vi "Determine Packet Type.vi"(11 "Packet First Byte":u8 format="%08b") -> (3 "Packet Type":refnum<class "ControlPacket.lvclass">)   [LabVIEW 2013, in "ControlPacket.lvclass"]
uses:
  ControlPacket.lvclass
  CONNECT/CONNECT.lvclass
  CONNACK/CONNACK.lvclass
  PUBLISH/PUBLISH.lvclass
  PUBACK/PUBACK.lvclass
  PUBREC/PUBREC.lvclass
  PUBREL/PUBREL.lvclass
  PUBCOMP/PUBCOMP.lvclass
  SUBSCRIBE/SUBSCRIBE.lvclass
  SUBACK/SUBACK.lvclass
  UNSUBSCRIBE/UNSUBSCRIBE.lvclass
  UNSUBACK/UNSUBACK.lvclass
  PINGREC/PINGREC.lvclass
  PINGRESP/PINGRESP.lvclass
  DISCONNECT/DISCONNECT.lvclass
  ControlPacket.lvclass/ControlPacket.ctl
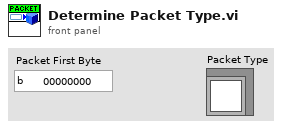
[diagram p1: front panel]
types:
  T1 = typedef "ControlPacket.lvclass/Control Packet Type -- enum.ctl" = enum16{"Reserved", "CONNECT", "CONNACK", "PUBLISH", "PUBACK", "PUBREC", "PUBREL", "PUBCOMP", "SUBSCRIBE", "SUBACK", "UNSUBSCRIBE", "UNSUBACK", "PINGREQ", "PINGRESP", "DISCONNECT", "Reserved(15)"}
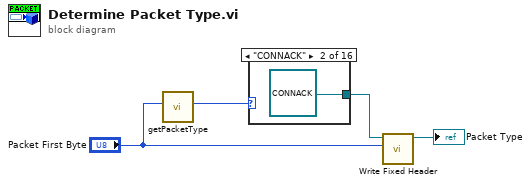
[diagram p0: block diagram]
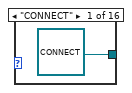
[diagram p2: hidden frame]
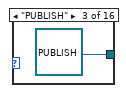
[diagram p3: hidden frame]
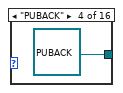
[diagram p4: hidden frame]
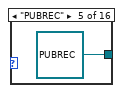
[diagram p5: hidden frame]
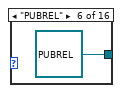
[diagram p6: hidden frame]
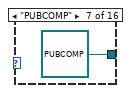
[diagram p7: hidden frame]
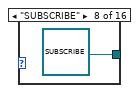
[diagram p8: hidden frame]
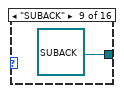
[diagram p9: hidden frame]
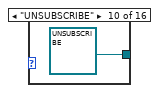
[diagram p10: hidden frame]
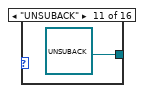
[diagram p11: hidden frame]
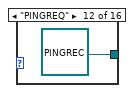
[diagram p12: hidden frame]
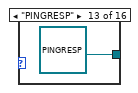
[diagram p13: hidden frame]
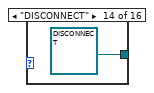
[diagram p14: hidden frame]
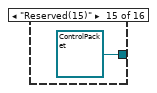
[diagram p15: hidden frame]
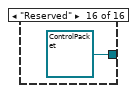
[diagram p16: hidden frame]
diagram:
  n1 = call "getPacketType.vi"("Packet First Byte"="Packet First Byte") -> ("Control Packet Type"=w1:T1)  [unwired: 10 in]
  n2 = case shown="\"CONNACK\"" w1 {
    tunnel: [refnum<class "CONNECT.lvclass"> refnum ("CONNECT.lvclass") refnum<class "CONNACK.lvclass"> refnum ("CONNACK.lvclass") refnum<class "PUBLISH.lvclass"> refnum ("PUBLISH.lvclass") refnum<class "PUBACK.lvclass"> refnum ("CONNECT.lvclass") refnum<class "PUBREC.lvclass"> refnum ("PUBREC.lvclass") refnum<class "PUBREL.lvclass"> refnum ("PUBREL.lvclass") refnum<class "PUBCOMP.lvclass"> refnum ("PUBCOMP.lvclass") refnum<class "SUBSCRIBE.lvclass"> refnum ("SUBSCRIBE.lvclass") refnum<class "SUBACK.lvclass"> refnum ("SUBACK.lvclass") refnum<class "UNSUBSCRIBE.lvclass"> refnum ("UNSUBSCRIBE.lvclass") refnum<class "UNSUBACK.lvclass"> refnum ("UNSUBACK.lvclass") refnum<class "PINGREC.lvclass"> refnum ("PINGREC.lvclass") refnum<class "PINGRESP.lvclass"> refnum ("PINGRESP.lvclass") refnum<class "DISCONNECT.lvclass"> refnum ("DISCONNECT.lvclass") refnum<class "ControlPacket.lvclass"> refnum ("CONNACK.lvclass") refnum<class "ControlPacket.lvclass"> refnum ("CONNACK.lvclass")] -> w3
    frame "CONNECT" {
    }
    frame "CONNACK" {
    }
    frame "PUBLISH" {
    }
    frame "PUBACK" {
    }
    frame "PUBREC" {
    }
    frame "PUBREL" {
    }
    frame "PUBCOMP" {
    }
    frame "SUBSCRIBE" {
    }
    frame "SUBACK" {
    }
    frame "UNSUBSCRIBE" {
    }
    frame "UNSUBACK" {
    }
    frame "PINGREQ" {
    }
    frame "PINGRESP" {
    }
    frame "DISCONNECT" {
    }
    frame "Reserved(15)" {
    }
    frame "Reserved" {
    }
  }
  n3 = call "Write Fixed Header.vi"("Fixed Header"="Packet First Byte", "ControlPacket in"=w3) -> ("ControlPacket out"=→"Packet Type":refnum<class "ControlPacket.lvclass">)  [unwired: 9 in]
